vi "Read Tag Class.vi"(2 "EnclaveChannel":T1) -> (7 "Lossy Reader":refnum<class "Tag.lvclass">, 9 "error out":errorcluster)   [LabVIEW 2022 SP3, in "Enclave.lvlib"]
uses:
  Enclave.lvlib
  ))Channel.ctl
  Element.ctl
  Tag/Tag.lvclass
  Operation.ctl
  Enclave/Enclave.lvclass
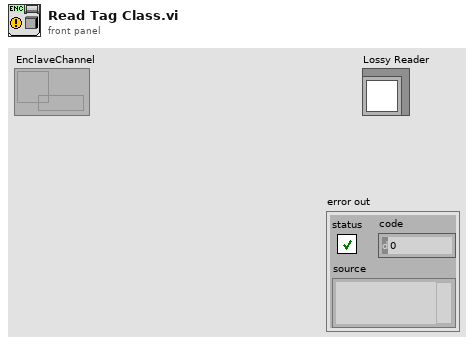
[diagram p1: front panel]
types:
  T1 = typedef "Enclave.lvlib/))Channel.ctl" = refnum<queue>
  T2 = typedef "Enclave.lvlib/Operation.ctl" = enum16{"Get Core", "Init", "Close"}
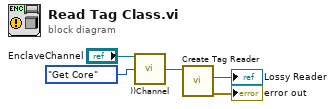
[diagram p0: block diagram]
diagram:
  n1 = call "))Channel.vi"("EnclaveChannel in"="EnclaveChannel", "Operation"=Operation."Get Core") -> ("Enclave"=w3:refnum<class "Enclave.lvclass">)  [unwired: 11 in, 2 out]
  n2 = call "Create Tag Reader.vi"("Enclave in"=w3) -> ("error out"=→"error out":errorcluster, "Lossy Reader"=→"Lossy Reader":refnum<class "Tag.lvclass">)  [unwired: 8 in, 1 out]
